vi "RT Driver_Display Debug String.vi"(8 "error in (no error)":errorcluster, 11 "Outputs In":dbl[](array[numeric])) -> (0 "error out":errorcluster)   [LabVIEW 2013, in "SNTP Light Custom Device Engine.lvlib"]
uses:
  SNTP Light Custom Device Engine.lvlib
  <vilib>/NI_Real-Time Target Support.lvlib
  <vilib>/NI Veristand/Custom Device Tools/Custom Device Utility Library/Custom Device Utility Library.lvlib
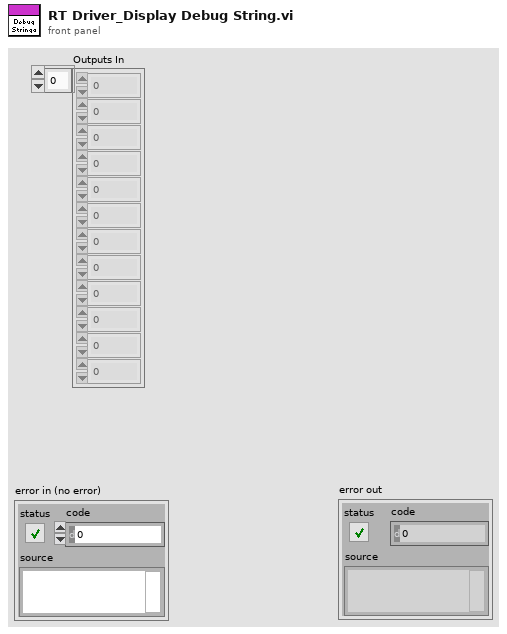
[diagram p1: front panel]
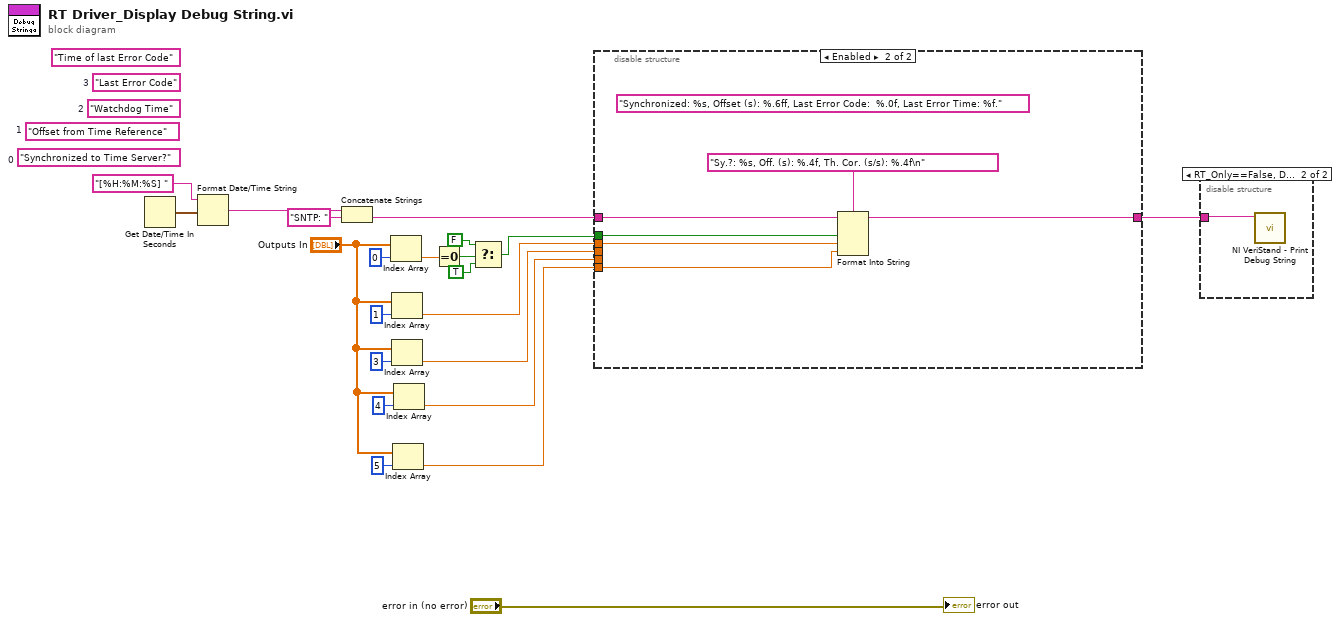
[diagram p0: block diagram]
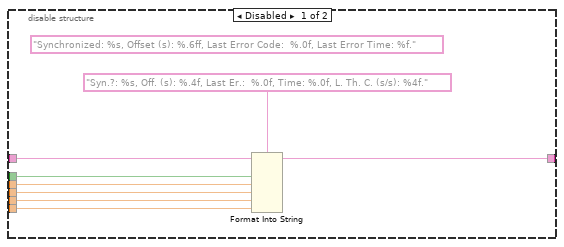
[diagram p2: hidden frame]
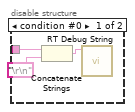
[diagram p3: hidden frame]
diagram:
  (unwired) "Time of last Error Code" ("Channel Name")
  (unwired) "Last Error Code"  # 3
  (unwired) "Watchdog Time"  # 2
  (unwired) "Offset from Time Reference"  # 1
  (unwired) "Synchronized to Time Server?"  # 0
  n1 = Get Date/Time In Seconds() -> (seconds since 1Jan1904=w5:timestamp)
  n2 = Format Date/Time String(time format string (%c)="[%H:%M:%S] ", seconds (now)=w5) -> (date/time string=w2:string)  [unwired: 1 in]
  n3 = Concatenate Strings(w2, "SNTP: " ("initial string")) -> (w1:string)
  n4 = Index Array(array="Outputs In", index=0) -> (element=w20:dbl)
  n5 = Index Array(array="Outputs In", index=1) -> (element=w14:dbl)
  n6 = Index Array(array="Outputs In", index=3) -> (element=w11:dbl)
  n7 = Index Array(array="Outputs In", index=5) -> (element=w6:dbl)
  n8 = Index Array(array="Outputs In", index=4) -> (element=w10:dbl)
  n9 = Equal To 0?(x=w20) -> (x = 0?=w19:bool)
  n10 = Select(t=FALSE, s=w19, f=TRUE) -> (s? t:f=w16:bool)
  n11 = disable-structure shown="Enabled" {
    disable-tunnel: w16 -> [w30 w36]
    disable-tunnel: w14 -> [w29 w35]
    disable-tunnel: w11 -> [w28 _]
    disable-tunnel: w10 -> [w27 _]
    disable-tunnel: [w26 w34] -> w9
    disable-tunnel: w6 -> [w24 w31]
    disable-tunnel: w1 -> [w23 w32]
    frame Disabled {
      (unwired) "Synchronized: %s, Offset (s): %.6ff, Last Error Code:  %.0f, Last Error Time: %f." ("format string")
      n12 = Format Into String(format string="Syn.?: %s, Off. (s): %.4f, Last Er.:  %.0f, Time: %.0f, L. Th. C. (s/s): %4f.", initial string=w23, w30, w29, w28, w27, w24) -> (resulting string=w26:string)  [unwired: 1 in, 1 out]
    }
    frame Enabled {
      (unwired) "Synchronized: %s, Offset (s): %.6ff, Last Error Code:  %.0f, Last Error Time: %f." ("format string")
      n13 = Format Into String(format string="Sy.?: %s, Off. (s): %.4f, Th. Cor. (s/s): %.4f\n", initial string=w32, w36, w35, w31) -> (resulting string=w34:string)  [unwired: 1 in, 1 out]
    }
  }
  n14 = disable-structure shown="RT_Only==False, Default" {
    disable-tunnel: w9 -> [w39 w40]
    frame condition #0 {
      n15 = Concatenate Strings(w39, "\r\n") -> (w38:string)
      n16 = call <vilib>:"RT Debug String.vi"("String to write"=w38) -> ()  [unwired: 10 in, 1 out]
    }
    frame condition #1 (active) {
      n17 = call <vilib>:"NI VeriStand - Print Debug String.vi"("Message"=w40) -> ()  [unwired: 10 in, 1 out]
    }
  }
  "error out" <- "error in (no error)"
